vi "Close FPGA Refs.vi"(8 "error in (no error)":errorcluster, 11 "FPGA Refs":T1 {"Data Type" format="%.0x"}) -> (0 "error out":errorcluster)   [LabVIEW 2015, in "Fuel Injector Analysis Addon Engine.lvlib"]
uses:
  Fuel Injector Analysis Addon Engine.lvlib
  Types/FPGA Refs.ctl
  Shared/Types/FPGA Data Types.ctl
  <vilib>/FPGAPlugInAG/Dynamic/niLvFpga_Close_Dynamic.vi
  <vilib>/rvi/interface/nirviCloseFPGA/nirviCloseFPGA.xnode
  Shared/Fuel Injector Analysis Addon Shared.lvlib
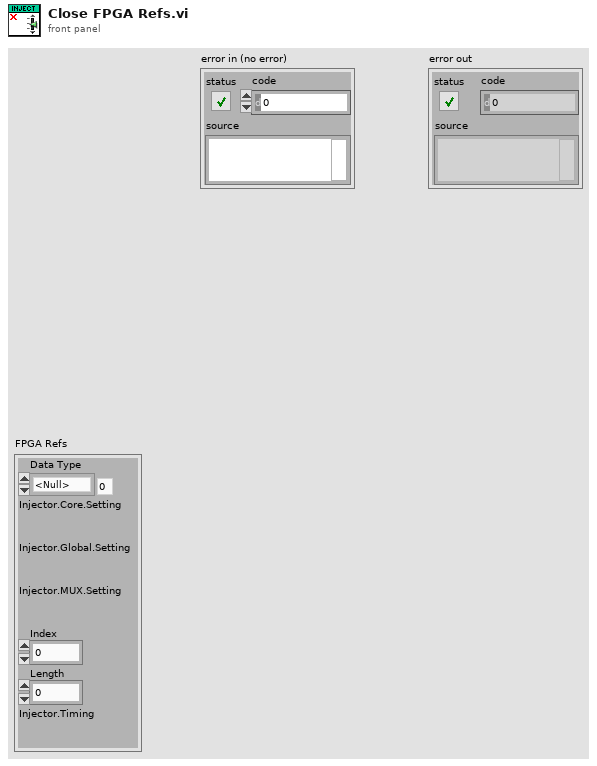
[diagram p1: front panel]
types:
  T1 = typedef "Fuel Injector Analysis Addon Engine.lvlib/FPGA Refs.ctl" = cluster{"Data Type":T2, "Injector.Core.Setting":refnum<k20>, "Injector.Global.Setting":refnum<k20>, "Injector.MUX.Setting":refnum<k20>, "Index":i32, "Length":i32, "Injector.Timing":refnum<k20>}
  T2 = typedef "Fuel Injector Analysis Addon Shared.lvlib/FPGA Data Types.ctl" = enum8{"<Null>", "Injector.Core.Setting", "Injector.Global.Setting", "Injector.Mux.Setting", "Injector.Timing"}
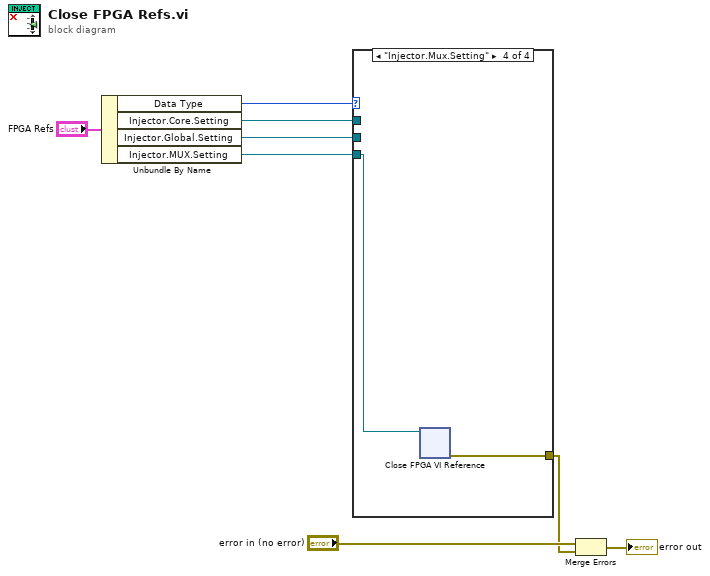
[diagram p0: block diagram]
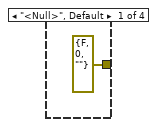
[diagram p2: hidden frame]
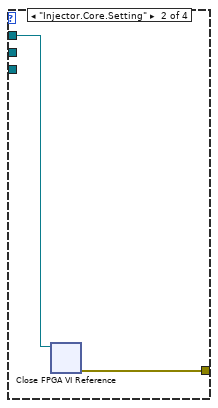
[diagram p3: hidden frame]
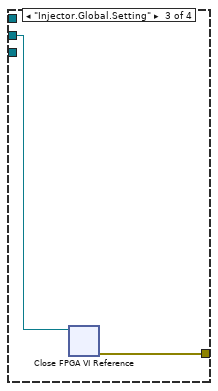
[diagram p4: hidden frame]
diagram:
  n1 = Unbundle By Name("FPGA Refs") -> ("Data Type"=w8:T2, "Injector.Core.Setting"=w4:refnum<k20>, "Injector.Global.Setting"=w5:refnum<k20>, "Injector.MUX.Setting"=w6:refnum<k20>)
  n2 = case shown="\"Injector.Mux.Setting\"" w8 {
    tunnel: [errorcluster {"status"=FALSE, "code"=0, "source"=""} ("error out") w11 w13 w15] -> w2
    tunnel: w6 -> [_ _ _ w14]
    tunnel: w5 -> [_ _ w12 _]
    tunnel: w4 -> [_ w10 _ _]
    frame "<Null>", Default {
    }
    frame "Injector.Core.Setting" {
      n3 = xnode "Close FPGA VI Reference"("FPGA VI Reference In"=w10) -> ("error out"=w11:errorcluster)  [unwired: 1 in]
    }
    frame "Injector.Global.Setting" {
      n4 = xnode "Close FPGA VI Reference"("FPGA VI Reference In"=w12) -> ("error out"=w13:errorcluster)  [unwired: 1 in]
    }
    frame "Injector.Mux.Setting" {
      n5 = xnode "Close FPGA VI Reference"("FPGA VI Reference In"=w14) -> ("error out"=w15:errorcluster)  [unwired: 1 in]
    }
  }
  n6 = Merge Errors("error in (no error)", w2) -> (→"error out":errorcluster)
